vi "Gen_Boolean.vi"(8 "error in (no error)":errorcluster) -> (0 "error out":errorcluster, 3 "Boolean":bool)   [LabVIEW 2015]
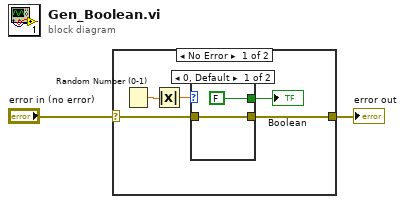
[diagram p0: block diagram]
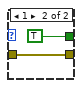
[diagram p2: hidden frame]
diagram:
  n1 = case shown="No Error" "error in (no error)" {
    selector: "error in (no error)" -> [w5 w12]
    tunnel: [w4 w12] -> w1
    frame No Error {
      n2 = Random Number (0-1)() -> (number: 0 to 1=w7:dbl)
      n3 = Absolute Value(x=w7) -> (abs(x)=w6:dbl)
      n4 = case shown="0, Default" w6 {
        tunnel: [w8 w11] -> w4
        tunnel: w5 -> [w8 w11]
        tunnel: [FALSE TRUE] -> w3
        frame 0, Default {
        }
        frame 1 {
        }
      }
      "Boolean" <- w3
    }
    frame Error {
    }
  }
  "error out" <- w1
